vi "File_FromEasyObj.vi"(8 "error in (no error)":errorcluster, 11 "output cluster":T1 {"Groups"."Channels"."Data Reference" format="%.0x"}) -> (0 "error out":errorcluster, 3 "File out":refnum<class "File.lvclass">)   [LabVIEW 2023, in "File.lvclass"]
doc: "Create a file class instance based on the given cluster of information defining the file, groups and channels."
uses:
  File.lvclass
  FileAsCluster.ctl
  Group/GroupAsCluster.ctl
  Channel/ChannelAsCluster.ctl
  <vilib>/NI VeriStand/Custom Device API/Data Reference.ctl
  Meta Data.ctl
  File.lvclass/File.ctl
  Group/Group.lvclass
  <vilib>/NI VeriStand/Custom Device API/Custom Device API.lvlib
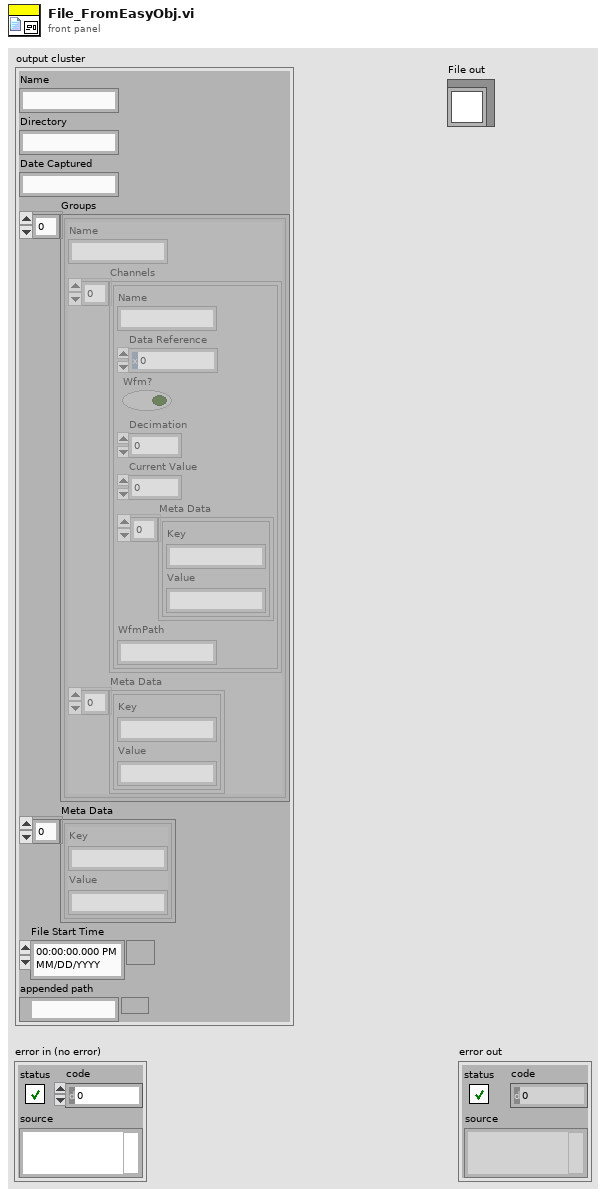
[diagram p1: front panel]
types:
  T1 = typedef "FileAsCluster.ctl" = cluster{"Name":string, "Directory":string, "Date Captured":string, "Groups":T2[], "Meta Data":T5[], "File Start Time":timestamp, "appended path":path}
  T2 = typedef "GroupAsCluster.ctl" = cluster{"Name":string, "Channels":T3[], "Meta Data":T5[]}
  T3 = typedef "ChannelAsCluster.ctl" = cluster{"Name":string, "Data Reference":T4, "Wfm?":bool, "Decimation":i32, "Current Value":dbl, "Meta Data":T5[], "WfmPath":string}
  T4 = typedef "Custom Device API.lvlib/Data Reference.ctl" = i32
  T5 = typedef "Meta Data.ctl" = cluster{"Key":string, "Value":string}
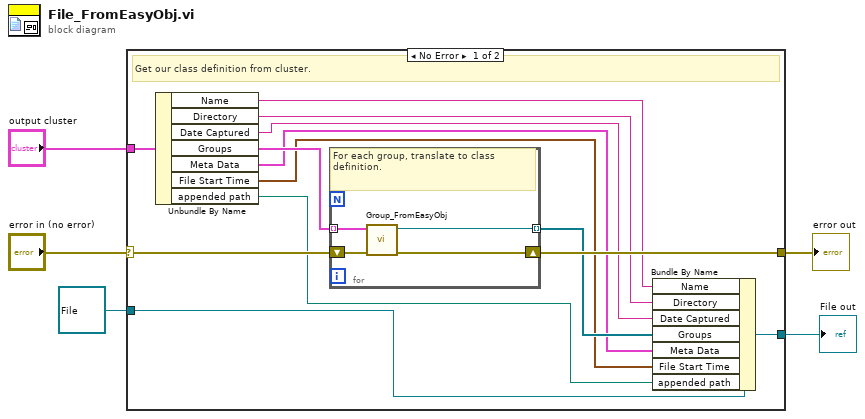
[diagram p0: block diagram]
diagram:
  n1 = case shown="No Error" "error in (no error)" {
    selector: "error in (no error)" -> [w14 w24]
    tunnel: [w13 w24] -> w4
    tunnel: [w16 w23] -> w2
    tunnel: refnum<class "File.lvclass"> refnum ("File in") -> [w17 w23]
    tunnel: "output cluster" -> [w18 _]
    frame No Error {
      # "Get our class definition from cluster."
      n2 = Unbundle By Name(w18) -> ("Name"=w6:string, "Directory"=w7:string, "Date Captured"=w8:string, "Groups"=w15:T2[], "Meta Data"=w11:T5[], "File Start Time"=w10:timestamp, "appended path"=w9:path)
      n3 = for {
        tunnel: w15 -> [w22] mode=indexing
        shift-right: [w20] -> w13
        shift-left: w14 -> [w21]
        tunnel: [w19] -> w12 mode=indexing
        # "For each group, translate to class definition."
        n4 = call "Group_FromEasyObj.vi"("error in (no error)"=w21, "input cluster"=w22) -> ("error out"=w20:errorcluster, "Group out"=w19:refnum<class "Group.lvclass">)  [unwired: 8 in]
      }
      n5 = Bundle By Name(cluster=w17, "Name"=w6, "Directory"=w7, "Date Captured"=w8, "Groups"=w12, "Meta Data"=w11, "File Start Time"=w10, "appended path"=w9) -> (w16:refnum<class "File.lvclass">)
    }
    frame Error {
    }
  }
  "error out" <- w4
  "File out" <- w2
